vi "Insert Key Value Pair (Nested).vi"(7 "key":string[](array[string]), 8 "error in (no error)":errorcluster, 10 "JSON Data in":refnum<class "JSON Datatype.lvclass">, 11 "JSON Object in":refnum<class "JSON Object.lvclass">) -> (0 "error out":errorcluster, 1 "replaced":bool, 3 "JSON Object Out":refnum<class "JSON Object.lvclass">)   [LabVIEW 2015, in "LVJSON.lvlib" / "JSON Object.lvclass"]
uses:
  JSON Object.lvclass
  JSON Datatype/JSON Datatype.lvclass
  JSON Datatype/To More Specific Type (Object).vi
  Insert Key Value Pair (Single).vi
  JSON Datatype/To More Specific Type (Array).vi
  JSON Array/Replace Array Subset (Single).vi
  JSON Array/JSON Array.lvclass
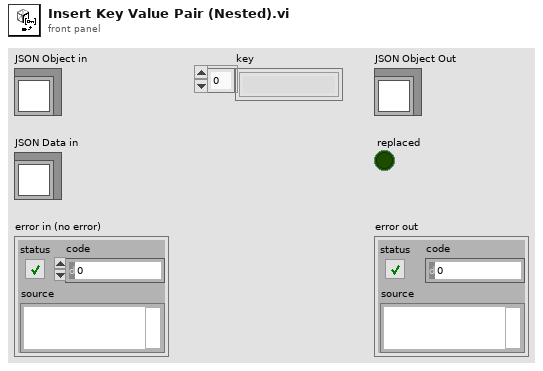
[diagram p1: front panel]
types:
  T1 = typedef "LVJSON.lvlib/JSON Types.ctl" = enum16{"String", "Numeric", "Boolean", "NULL", "Object", "Array", "Unknown"}
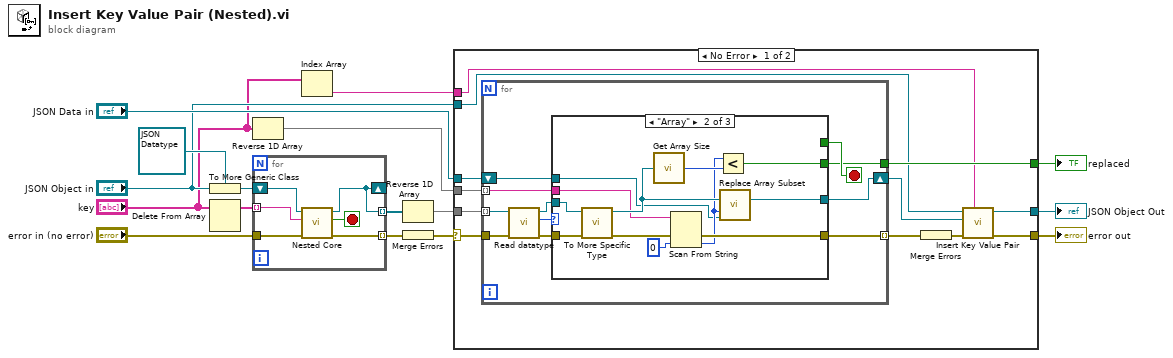
[diagram p0: block diagram]
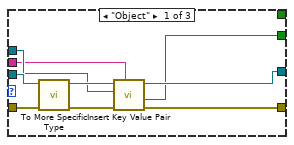
[diagram p2: hidden frame]
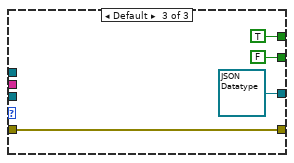
[diagram p3: hidden frame]
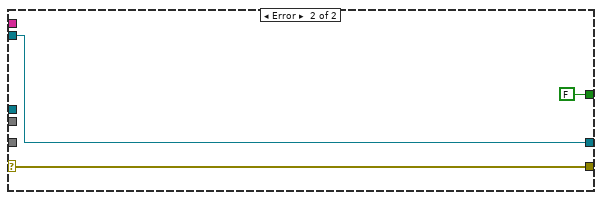
[diagram p4: hidden frame]
diagram:
  n1 = To More Generic Class(target class=refnum<class "JSON Datatype.lvclass"> refnum, reference="JSON Object in") -> (generic class reference=w8:refnum<class "JSON Datatype.lvclass">)
  n2 = Delete From Array(array="key") -> (array with subset deleted=w12:string[])  [unwired: 2 in, 1 out]
  n3 = Reverse 1D Array(array="key") -> (reversed array=w13:string[])
  n4 = for {
    tunnel: w12 -> [w22] mode=indexing
    shift-right: [w17] -> _
    shift-left: w8 -> [w21]
    tunnel: "error in (no error)" -> [w20]
    tunnel: [w19] -> w9 mode=indexing
    tunnel: [w17] -> w10 mode=indexing
    stop <- w18 stop-if-true
    n5 = call "Nested Core.vi"("error in (no error)"=w20, "key"=w22, "JSON Datatype in"=w21) -> ("error out"=w19:errorcluster, "stop?"=w18:bool, "JSON Datatype out"=w17:refnum<class "JSON Datatype.lvclass">)  [unwired: 5 in, 1 out]
  }
  n6 = Index Array(array="key") -> (element=w1:string)  [unwired: 1 in]
  n7 = Reverse 1D Array(array=w10) -> (reversed array=w14:refnum<class "JSON Datatype.lvclass">[])
  n8 = Merge Errors(w9) -> (w11:errorcluster)
  n9 = case shown="No Error" w11 {
    selector: w11 -> [w30 w71]
    tunnel: [w34 FALSE ("replaced")] -> w16
    tunnel: "JSON Data in" -> [w33 _]
    tunnel: w14 -> [w32 _]
    tunnel: w13 -> [w31 _]
    tunnel: [w26 w73] -> w4
    tunnel: "JSON Object in" -> [w28 w73]
    tunnel: [w24 w71] -> w3
    tunnel: w1 -> [w23 _]
    frame No Error {
      n10 = for {
        tunnel: w31 -> [w37] mode=indexing
        tunnel: w30 -> [w43]
        tunnel: [w42] -> w29 mode=indexing
        tunnel: [w39] -> w34
        tunnel: w32 -> [w38] mode=indexing
        shift-right: [w36] -> w27
        shift-left: w33 -> [w35]
        stop <- w40 stop-if-true
        n11 = call-dynamic "Read datatype.vi"("error in (no error)"=w43, "JSON Datatype in"=w38) -> ("error out"=w41:errorcluster, "datatype"=w44:T1, "JSON Datatype out"=w45:refnum<class "JSON Datatype.lvclass">)  [unwired: 7 in]
        n12 = case shown="\"Array\"" w44 {
          tunnel: w37 -> [w46 w55 _]
          tunnel: [w48 w57 refnum<class "JSON Datatype.lvclass"> refnum ("JSON Data")] -> w36
          tunnel: w45 -> [w53 w66 _]
          tunnel: [w50 w62 w68] -> w42
          tunnel: w41 -> [w52 w64 w68]
          tunnel: [_ _ TRUE] -> w40
          tunnel: [w47 w58 FALSE] -> w39
          tunnel: w35 -> [w49 w56 _]
          frame "Object" {
            n13 = call-poly "To More Specific Type.vi"("error in (no error)"=w52, "JSON Datatype in"=w53) -> ("error out"=w51:errorcluster, "JSON Datatype out"=w54:refnum<class "JSON Object.lvclass">)  [unwired: 8 in]
            n14 = call-poly "Insert Key Value Pair.vi"("key"=w46, "error in (no error)"=w51, "value"=w49, "JSON Object in"=w54) -> ("error out"=w50:errorcluster, "replaced"=w47:bool, "JSON Object out"=w48:refnum<class "JSON Object.lvclass">)  [unwired: 5 in]
          }
          frame "Array" {
            n15 = call-poly "To More Specific Type.vi"("error in (no error)"=w64, "JSON Datatype in"=w66) -> ("error out"=w63:errorcluster, "JSON Datatype out"=w61:refnum<class "JSON Array.lvclass">)  [unwired: 8 in]
            n16 = call "Get Array Size.vi"("JSON Array in"=w61) -> ("size(s)"=w60:i32)
            n17 = Scan From String(input string=w55, error in=w63, default 1=0 ("index")) -> (error out=w62:errorcluster, output 1=w59:i32)  [unwired: 2 in, 2 out]
            n18 = Less?(x=w59, y=w60) -> (x < y?=w58:bool)
            n19 = call-poly "Replace Array Subset.vi"("JSON Array"=w61, "index"=w59, "new element/subarray"=w56) -> ("output JSON Array"=w57:refnum<class "JSON Array.lvclass">)  [unwired: 12 in]
          }
          frame Default {
          }
        }
      }
      n20 = Merge Errors(w29) -> (w25:errorcluster)
      n21 = call-poly "Insert Key Value Pair.vi"("key"=w23, "error in (no error)"=w25, "value"=w27, "JSON Object in"=w28) -> ("error out"=w24:errorcluster, "JSON Object out"=w26:refnum<class "JSON Object.lvclass">)  [unwired: 5 in, 1 out]
    }
    frame Error {
    }
  }
  "replaced" <- w16
  "error out" <- w3
  "JSON Object Out" <- w4
